vi "Main_Sub_Trigger.vi"(7 "Trigger_Action":enum16{"Initial", "Set"}(ring), 11 "Trigger":bool) -> (3 "Trigger_Action Out":T1)   [LabVIEW 2015]
uses:
  1.Control/Control_Main_Trigger Action Out.ctl
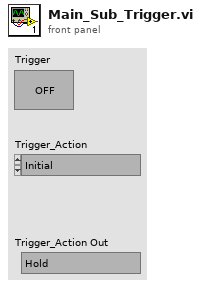
[diagram p1: front panel]
types:
  T1 = typedef "Control_Main_Trigger Action Out.ctl" = enum16{"Hold", "Stop", "Start"}
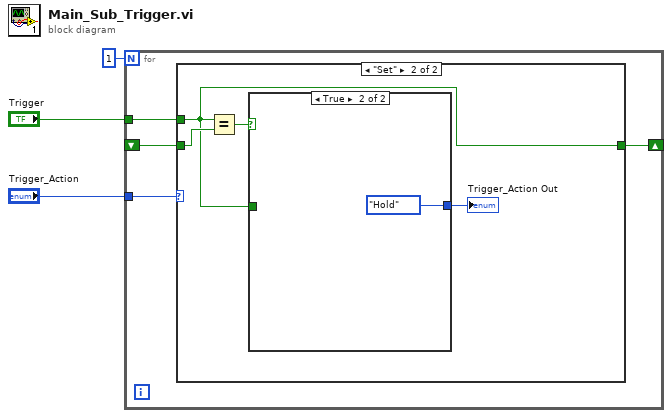
[diagram p0: block diagram]
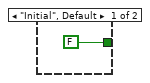
[diagram p2: hidden frame]
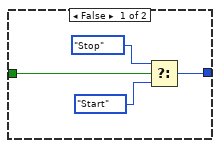
[diagram p3: hidden frame]
diagram:
  n1 = for {
    N: 1 -> [_]
    tunnel: "Trigger" -> [w5]
    shift-right: [w6] -> _
    shift-left: _ -> [w4]
    tunnel: "Trigger_Action" -> [w7]
    n2 = case shown="\"Set\"" w7 {
      tunnel: [FALSE w9] -> w6
      tunnel: w5 -> [_ w9]
      tunnel: w4 -> [_ w12]
      frame "Initial", Default {
      }
      frame "Set" {
        n3 = Equal?(x=w9, y=w12) -> (x = y?=w11:bool)
        n4 = case shown="True" w11 {
          tunnel: w9 -> [w16 _]
          tunnel: [w13 Control_Main_Trigger_Action_Out."Hold" ("Trigger_Action Out")] -> w10
          frame False {
            n5 = Select(t=Control_Main_Trigger_Action_Out."Stop" ("Trigger_Action Out"), s=w16, f=Control_Main_Trigger_Action_Out."Start" ("Trigger_Action Out")) -> (s? t:f=w13:T1)
          }
          frame True {
          }
        }
        "Trigger_Action Out" <- w10
      }
    }
  }
